vi "MainUseLVOOP.vi"() -> ()   [LabVIEW 2021]
uses:
  ClassicType/ClassicType.lvclass
  C:/Users/chrismadlax/Documents/LabVIEW Data/Project/OOP/GeneralCar/GeneralCar.lvclass
  LuxuryType/LuxuryType.lvclass
  GeneralCar/GeneralCar.lvclass/GeneralCar.ctl
  GeneralCar/GeneralCar.lvclass
panel:
  out "生產資訊":string
  in  "車型":enum16{"經典", "加長豪華"}(ring)
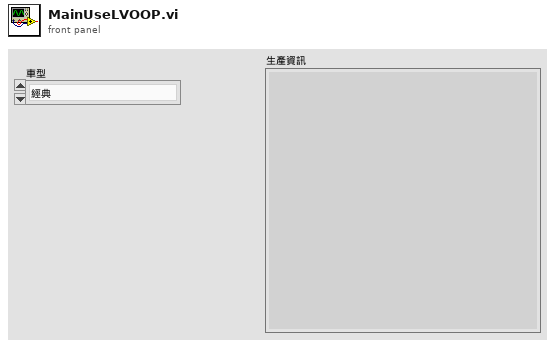
[diagram p1: front panel]
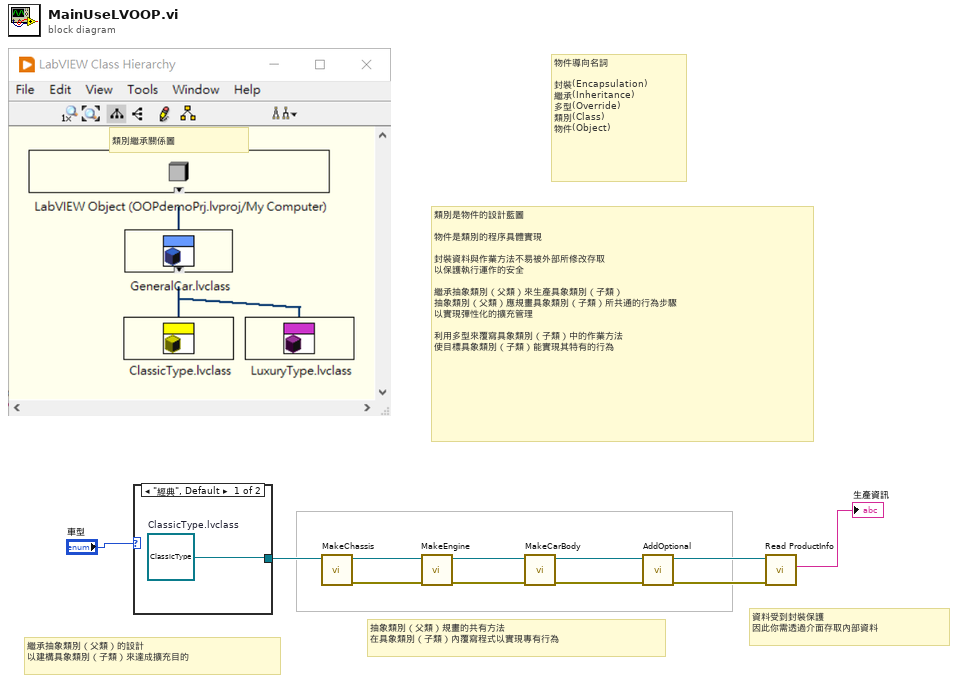
[diagram p0: block diagram]
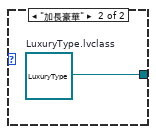
[diagram p2: hidden frame]
diagram:
  # "類別繼承關係圖"
  # "繼承抽象類別（父類）的設計\n以建構具象類別（子類）來達成擴充目的"
  # "抽象類別（父類）規畫的共有方法\n在具象類別（子類）內覆寫程式以實現專有行為"
  # "資料受到封裝保護\n因此你需透過介面存取內部資料"
  # "物件導向名詞\n\n封裝(Encapsulation)\n繼承(Inheritance)\n多型(Override)\n類別(Class)\n物件(Object)"
  # "類別是物件的設計藍圖\n\n物件是類別的程序具體實現\n\n封裝資料與作業方法不易被外部所修改存取\n以保護執行運作的安全\n\n繼承抽象類別（父類）來生產具象類別（子類）\n抽象類別（父類）應規畫具象類別（子類）所共通的行為步驟\n以實現彈性化的擴充管理\n\n利用多型來覆寫具象類別（子類）中的作業方法\n使目標具象類別（子類）能實現其特有的行為"
  n1 = case shown="\"經典\", Default" "車型" {
    tunnel: [w12 w13] -> w4
    frame "經典", Default {
      w12 = refnum<class "ClassicType.lvclass"> refnum  # ClassicType.lvclass
    }
    frame "加長豪華" {
      w13 = refnum<class "LuxuryType.lvclass"> refnum  # LuxuryType.lvclass
    }
  }
  n2 = call-dynamic "MakeChassis.vi"("GeneralCar in"=w4) -> ("error out"=w5:errorcluster, "GeneralCar out"=w6:refnum<class "GeneralCar.lvclass">)  [unwired: 9 in]
  n3 = call-dynamic "MakeEngine.vi"("error in (no error)"=w5, "GeneralCar in"=w6) -> ("error out"=w9:errorcluster, "GeneralCar out"=w10:refnum<class "GeneralCar.lvclass">)  [unwired: 8 in]
  n4 = call-dynamic "MakeCarBody.vi"("error in (no error)"=w9, "GeneralCar in"=w10) -> ("error out"=w7:errorcluster, "GeneralCar out"=w8:refnum<class "GeneralCar.lvclass">)  [unwired: 8 in]
  n5 = call-dynamic "AddOptional.vi"("error in (no error)"=w7, "GeneralCar in"=w8) -> ("error out"=w2:errorcluster, "GeneralCar out"=w3:refnum<class "GeneralCar.lvclass">)  [unwired: 8 in]
  n6 = call "Read ProductInfo.vi"("error in (no error)"=w2, "GeneralCar in"=w3) -> ("ProductInfo"=→"生產資訊":string)  [unwired: 7 in, 2 out]
